vi "Top (FPGA).vi"() -> ()   [LabVIEW 2024, in "PXIe-7903 Aurora Example.lvlib"]
uses:
  PXIe-7903 Aurora Example.lvlib
  <vilib>/Platform/TimedLoop/XDataNode/wakeup.ctl
  <vilib>/Platform/TimedLoop/XDataNode/XDNodeRunTimeDep.lvlib
  <vilib>/Platform/TimedLoop/XDataNode/nitl_modes.ctl
  <vilib>/Platform/TimedLoop/XDataNode/timing_clust.ctl
  <vilib>/Platform/TimedLoop/XDataNode/XDataNode.xnode
  <instrlib>/_niInstr/FIFO Register Bus/v1/FPGA/niInstr FIFO Register Bus v1 FPGA.lvclass
  <instrlib>/_niInstr/Instruction Framework/v1/FPGA/Top Level Bus/Register Configuration/Register Configuration.lvclass
  <instrlib>/_niInstr/Instruction Framework/v1/FPGA/Collection Builder/Collection Builder.lvclass
  <instrlib>/_niInstr/Instruction Framework/v1/FPGA/Collection Builder/Parent Metadata.ctl
  <instrlib>/_niInstr/Instruction Framework/v1/FPGA/Collection Builder/niInstr Address Space Collection Builder v1 FPGA.lvlib
  <vilib>/eio/EIONode/EIONode.xnode
  Utilities/FPGA/Aurora64b66b Utilities FPGA.lvlib
  <instrlib>/_niInstr/Basic Elements/v1/FPGA/niInstr Basic Elements v1 FPGA.lvlib
  <vilib>/rvi/eio/common/nirviEmuTemplateMethod_errors.vi
  <instrlib>/_niInstr/Aurora64b66b/v1/FPGA/Buffered/Aurora64b66b Buffered.lvclass
panel:
  in  "port 11 enable":bool
  in  "port 10 enable":bool
  in  "port 9 enable":bool
  in  "port 8 enable":bool
  in  "port 7 enable":bool
  in  "port 6 enable":bool
  in  "port 5 enable":bool
  in  "port 4 enable":bool
  in  "port 3 enable":bool
  in  "port 2 enable":bool
  in  "port 1 enable":bool
  in  "port 0 enable":bool
  in  "port 11 rx throttle":u16
  out "port 11 mismatch count":u64
  in  "port 10 rx throttle":u16
  out "port 10 mismatch count":u64
  in  "port 9 rx throttle":u16
  out "port 9 mismatch count":u64
  in  "port 8 rx throttle":u16
  out "port 8 mismatch count":u64
  in  "port 7 rx throttle":u16
  out "port 7 mismatch count":u64
  in  "port 6 rx throttle":u16
  out "port 6 mismatch count":u64
  in  "port 5 rx throttle":u16
  out "port 5 mismatch count":u64
  in  "port 4 rx throttle":u16
  out "port 4 mismatch count":u64
  in  "port 3 rx throttle":u16
  out "port 3 mismatch count":u64
  in  "port 2 rx throttle":u16
  out "port 2 mismatch count":u64
  in  "port 1 rx throttle":u16
  out "port 1 mismatch count":u64
  out "port 0 mismatch count":u64
  in  "port 0 rx throttle":u16
  in  "tb reset":bool
  out "flexrio.module.io error 0":i32
  out "flexrio.module.io ready 0":bool
  in  "fifo reg bus ctrl 0":u32
  out "fifo reg bus status 0":u32
  out "fifo reg bus data 0":u64
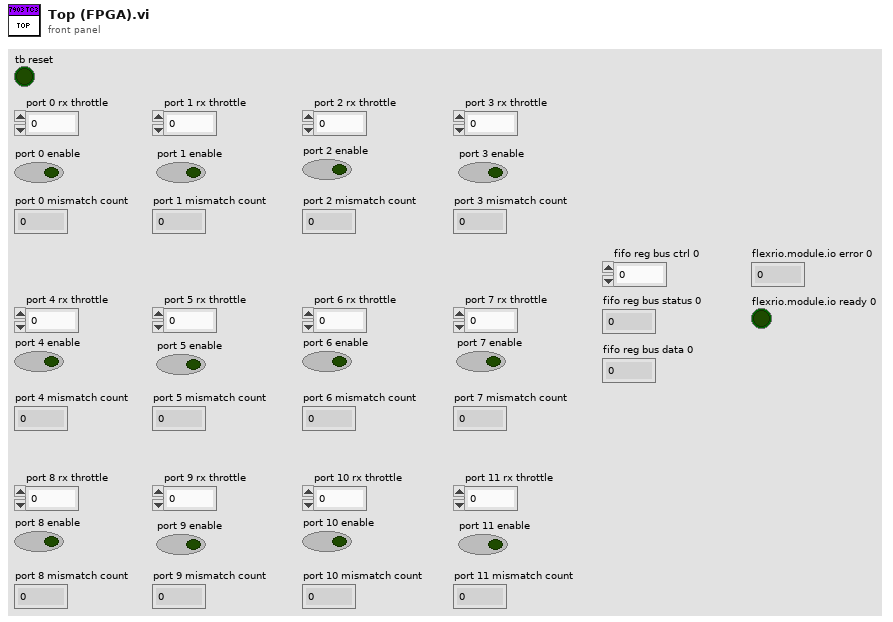
[diagram p1: front panel]
types:
  T1 = typedef "niInstr Address Space Collection Builder v1 FPGA.lvlib/Parent Metadata.ctl" = cluster{"UID":u16, "version":u16, "oldest compatible version":u16}
  T2 = typedef "XDNodeRunTimeDep.lvlib/timing_clust.ctl" = cluster{"Expected End [f-1]":u64, "Actual End [f-1]":u64, "Finished Late? [f-1]":bool, "Expected End [i-1]":u64, "Actual End [i-1]":u64, "Finished Late? [i-1]":bool, "Expected Start [i]":u64, "Actual Start [i]":u64, "Expected Start [f]":u64, "Actual Start [f]":u64, "Source Name":string, "Structure Name":string, "Period":i64, "Deadline":i64, "Offset":i64, "Start":i64, "Priority":i32, "Timeout":i32, "Mode":T3, "Wakeup Reason":T4, "Error":errorcluster, "Source Type":string, "Secondary Source Type":string, "Global End Time":u64, "Global Start Time":u64, "Frame Duration":u64, "Iteration Duration":u64, "Assigned CPU":i32, "I/O Scan Engine Mode":u32}
  T3 = typedef "XDNodeRunTimeDep.lvlib/nitl_modes.ctl" = enum32{"No Change", "Process missed periods, maintain original phase", "Discard missed periods, maintain original phase", "Process missed periods, ignore original phase", "Discard missed periods, ignore original phase"}
  T4 = typedef "XDNodeRunTimeDep.lvlib/wakeup.ctl" = enum32{"Normal", "Aborted", "Asynchronous wakeup", "Timing source error", "Timed loop error", "Timeout"}
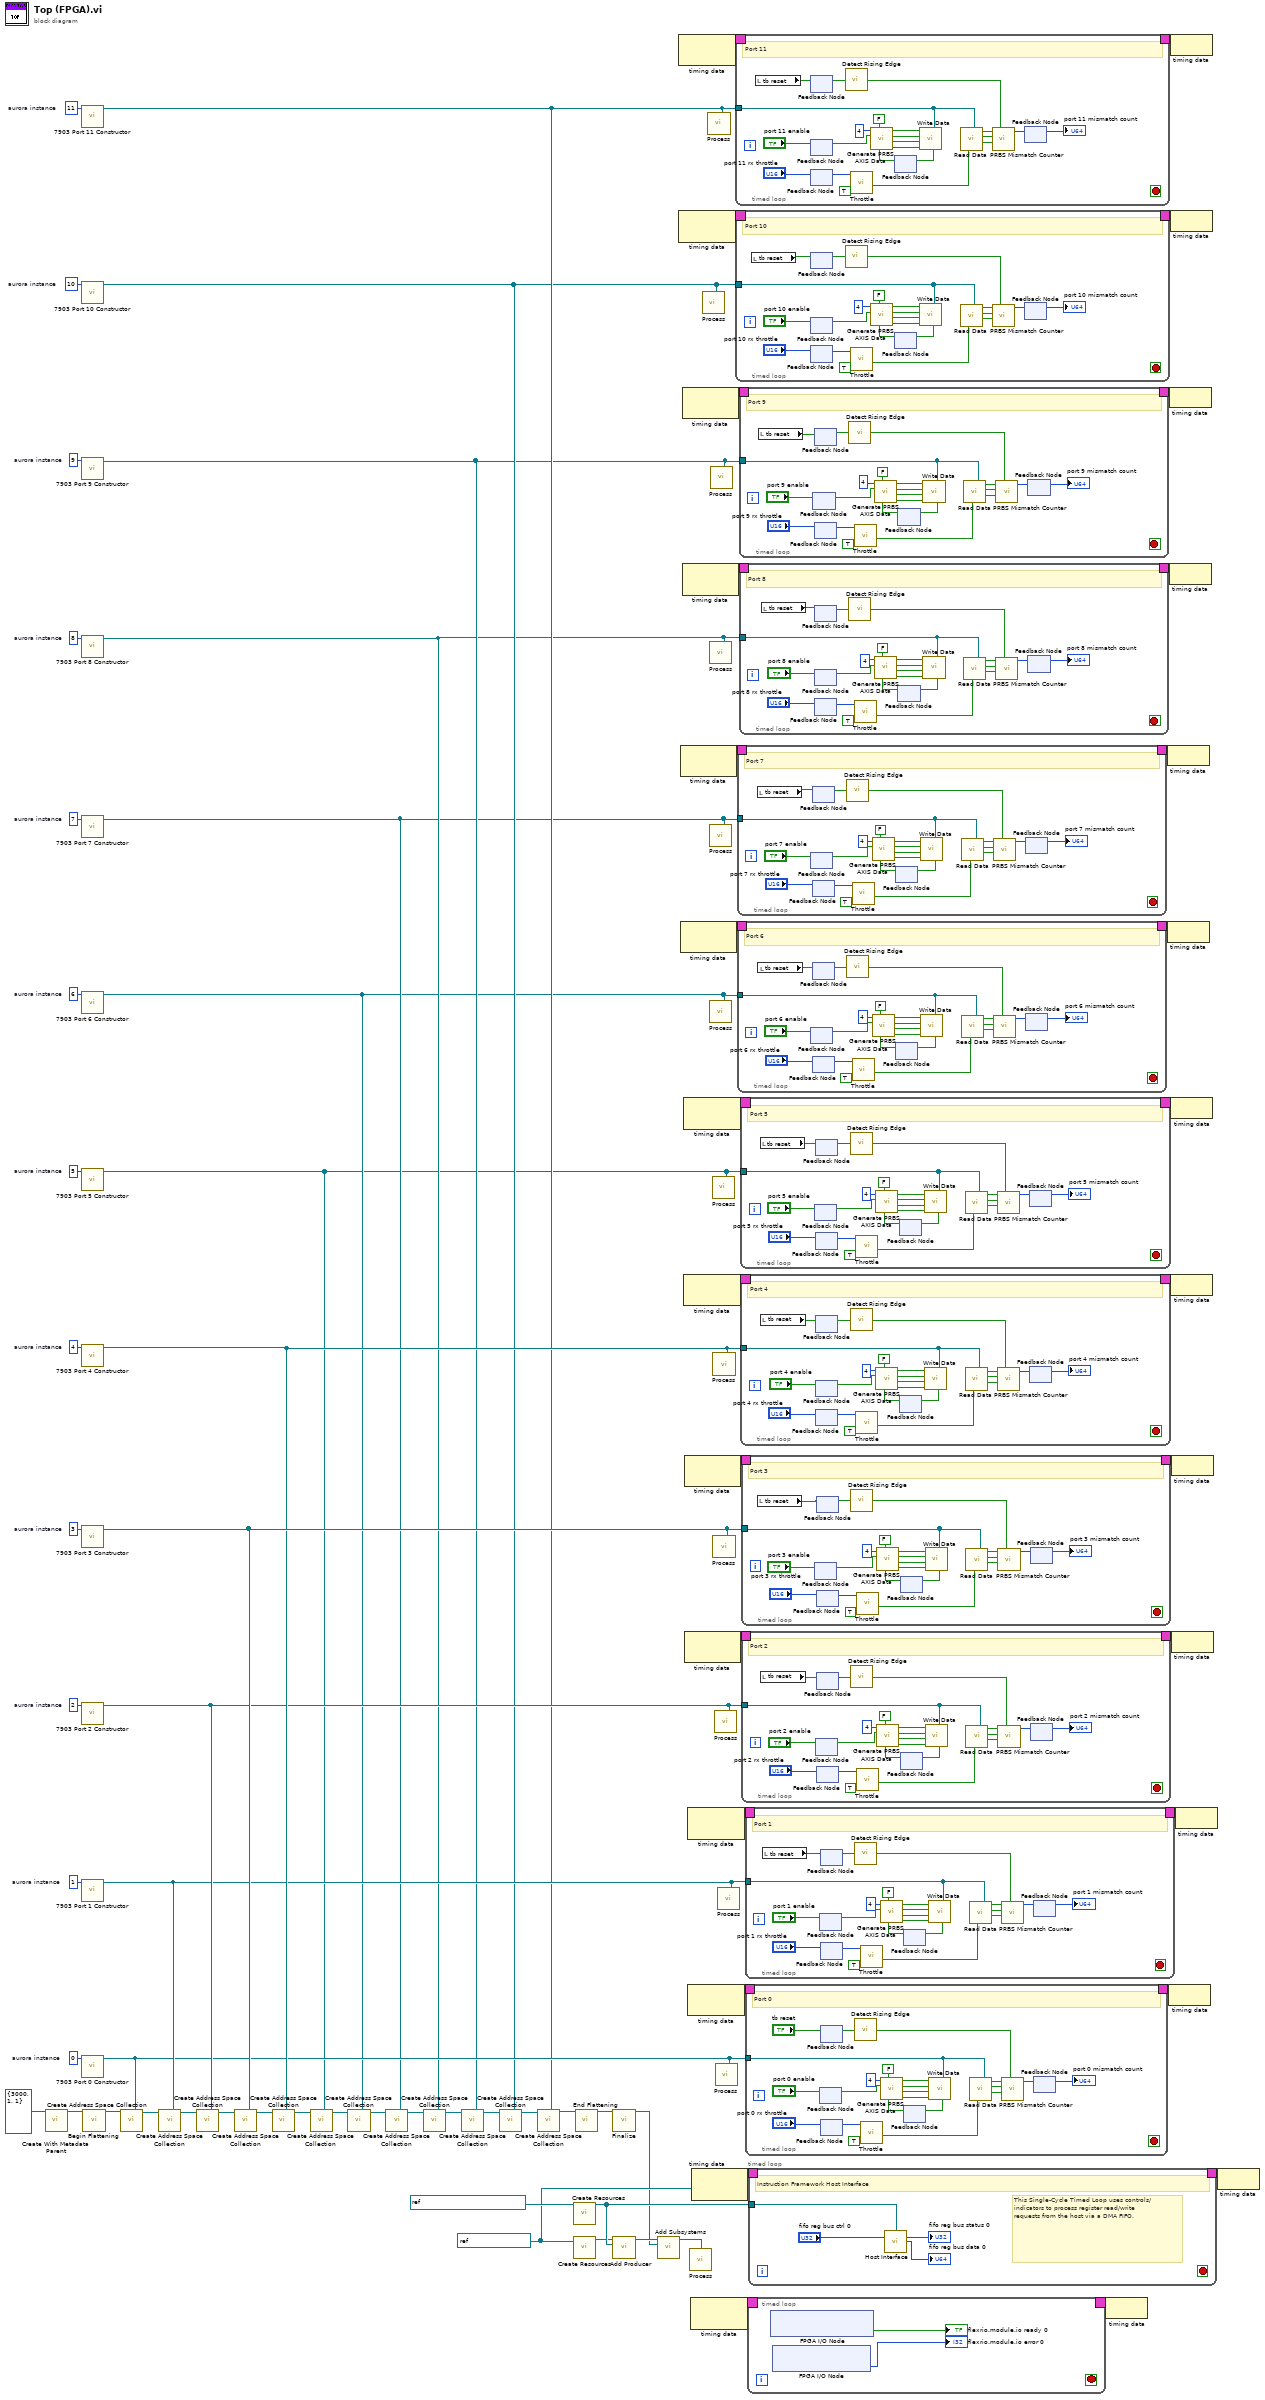
[diagram p0: block diagram]
diagram:
  w1 = u8 11  # aurora instance
  w48 = u8 10  # aurora instance
  w49 = u8 9  # aurora instance
  w50 = u8 8  # aurora instance
  w51 = u8 3  # aurora instance
  w52 = u8 2  # aurora instance
  w53 = u8 1  # aurora instance
  w54 = u8 0  # aurora instance
  w56 = u8 7  # aurora instance
  w57 = u8 6  # aurora instance
  w58 = u8 5  # aurora instance
  w59 = u8 4  # aurora instance
  w70 = refnum<k21> "80 MHz Clock" ("Source Name")
  n1 = call <instrlib>:"Create With Metadata Parent.vi"("parent metadata"=T1 {"UID"=3000, "version"=1, "oldest compatible version"=1}) -> ("collection builder"=w69:refnum<class "Collection Builder.lvclass">)  [unwired: 14 in]
  n2 = call "7903 Port 11 Constructor.vi"("aurora instance (0)"=w1) -> ("aurora64b66b buffered"=w8:refnum<class "Aurora64b66b Buffered.lvclass">)  [unwired: 10 in]
  n3 = call "7903 Port 10 Constructor.vi"("aurora instance (0)"=w48) -> ("aurora64b66b buffered"=w7:refnum<class "Aurora64b66b Buffered.lvclass">)  [unwired: 10 in]
  n4 = call "7903 Port 9 Constructor.vi"("aurora instance (0)"=w49) -> ("aurora64b66b buffered"=w6:refnum<class "Aurora64b66b Buffered.lvclass">)  [unwired: 10 in]
  n5 = call "7903 Port 8 Constructor.vi"("aurora instance (0)"=w50) -> ("aurora64b66b buffered"=w5:refnum<class "Aurora64b66b Buffered.lvclass">)  [unwired: 10 in]
  n6 = call "7903 Port 7 Constructor.vi"("aurora instance (0)"=w56) -> ("aurora64b66b buffered"=w4:refnum<class "Aurora64b66b Buffered.lvclass">)  [unwired: 10 in]
  n7 = call "7903 Port 6 Constructor.vi"("aurora instance (0)"=w57) -> ("aurora64b66b buffered"=w3:refnum<class "Aurora64b66b Buffered.lvclass">)  [unwired: 10 in]
  n8 = call "7903 Port 5 Constructor.vi"("aurora instance (0)"=w58) -> ("aurora64b66b buffered"=w2:refnum<class "Aurora64b66b Buffered.lvclass">)  [unwired: 10 in]
  n9 = call "7903 Port 4 Constructor.vi"("aurora instance (0)"=w59) -> ("aurora64b66b buffered"=w12:refnum<class "Aurora64b66b Buffered.lvclass">)  [unwired: 10 in]
  n10 = call "7903 Port 3 Constructor.vi"("aurora instance (0)"=w51) -> ("aurora64b66b buffered"=w13:refnum<class "Aurora64b66b Buffered.lvclass">)  [unwired: 10 in]
  n11 = call "7903 Port 2 Constructor.vi"("aurora instance (0)"=w52) -> ("aurora64b66b buffered"=w11:refnum<class "Aurora64b66b Buffered.lvclass">)  [unwired: 10 in]
  n12 = call "7903 Port 1 Constructor.vi"("aurora instance (0)"=w53) -> ("aurora64b66b buffered"=w10:refnum<class "Aurora64b66b Buffered.lvclass">)  [unwired: 10 in]
  n13 = call "7903 Port 0 Constructor.vi"("aurora instance (0)"=w54) -> ("aurora64b66b buffered"=w9:refnum<class "Aurora64b66b Buffered.lvclass">)  [unwired: 10 in]
  n14 = call <instrlib>:"Begin Flattening.vi"("collection builder in"=w69) -> ("collection builder out"=w63:refnum<class "Collection Builder.lvclass">)  [unwired: 14 in]
  n15 = call-dynamic "Create Address Space Collection.vi"("aurora64b66b basic"=w9, "collection builder in"=w63) -> ("collection builder out"=w55:refnum<class "Collection Builder.lvclass">)  [unwired: 9 in]
  n16 = call-dynamic "Create Address Space Collection.vi"("aurora64b66b basic"=w10, "collection builder in"=w55) -> ("collection builder out"=w41:refnum<class "Collection Builder.lvclass">)  [unwired: 9 in]
  n17 = call-dynamic "Create Address Space Collection.vi"("aurora64b66b basic"=w11, "collection builder in"=w41) -> ("collection builder out"=w42:refnum<class "Collection Builder.lvclass">)  [unwired: 9 in]
  n18 = call-dynamic "Create Address Space Collection.vi"("aurora64b66b basic"=w13, "collection builder in"=w42) -> ("collection builder out"=w47:refnum<class "Collection Builder.lvclass">)  [unwired: 9 in]
  n19 = call-dynamic "Create Address Space Collection.vi"("aurora64b66b basic"=w12, "collection builder in"=w47) -> ("collection builder out"=w46:refnum<class "Collection Builder.lvclass">)  [unwired: 9 in]
  n20 = call-dynamic "Create Address Space Collection.vi"("aurora64b66b basic"=w2, "collection builder in"=w46) -> ("collection builder out"=w45:refnum<class "Collection Builder.lvclass">)  [unwired: 9 in]
  n21 = call-dynamic "Create Address Space Collection.vi"("aurora64b66b basic"=w3, "collection builder in"=w45) -> ("collection builder out"=w44:refnum<class "Collection Builder.lvclass">)  [unwired: 9 in]
  n22 = call-dynamic "Create Address Space Collection.vi"("aurora64b66b basic"=w4, "collection builder in"=w44) -> ("collection builder out"=w43:refnum<class "Collection Builder.lvclass">)  [unwired: 9 in]
  n23 = call-dynamic "Create Address Space Collection.vi"("aurora64b66b basic"=w5, "collection builder in"=w43) -> ("collection builder out"=w38:refnum<class "Collection Builder.lvclass">)  [unwired: 9 in]
  n24 = call-dynamic "Create Address Space Collection.vi"("aurora64b66b basic"=w6, "collection builder in"=w38) -> ("collection builder out"=w40:refnum<class "Collection Builder.lvclass">)  [unwired: 9 in]
  n25 = call-dynamic "Create Address Space Collection.vi"("aurora64b66b basic"=w7, "collection builder in"=w40) -> ("collection builder out"=w39:refnum<class "Collection Builder.lvclass">)  [unwired: 9 in]
  n26 = call-dynamic "Create Address Space Collection.vi"("aurora64b66b basic"=w8, "collection builder in"=w39) -> ("collection builder out"=w60:refnum<class "Collection Builder.lvclass">)  [unwired: 9 in]
  n27 = call <instrlib>:"Create Resources.vi"("instruction fifo"=refnum<k21> "reg.host instruction fifo 0" ("FIFO")) -> ("fifo register bus"=w72:refnum<class "niInstr FIFO Register Bus v1 FPGA.lvclass">)  [unwired: 14 in]
  n28 = call <instrlib>:"Create Resources.vi"("register clock"=w70) -> ("register configuration"=w71:refnum<class "Register Configuration.lvclass">)  [unwired: 14 in]
  n29 = call <instrlib>:"End Flattening.vi"("collection builder in"=w60) -> ("collection builder out"=w68:refnum<class "Collection Builder.lvclass">)  [unwired: 14 in]
  n30 = call <instrlib>:"Finalize.vi"("collection builder in"=w68) -> ("address space collection"=w64:refnum<class "Address Space Collection.lvclass">)  [unwired: 14 in]
  n31 = call-dynamic "Add Producer.vi"("register configuration in"=w71, "instruction producer"=w72) -> ("register configuration out"=w66:refnum<class "Register Configuration.lvclass">)  [unwired: 13 in]
  n32 = call-dynamic "Add Subsystems.vi"("register configuration in"=w66, "subsystems"=w64) -> ("register configuration out"=w65:refnum<class "Register Configuration.lvclass">)  [unwired: 13 in]
  n33 = node-c288() -> (w15:T2)  [unwired: 1 in]
  n34 = node-c288() -> (w17:T2)  [unwired: 1 in]
  n35 = node-c288() -> (w23:T2)  [unwired: 1 in]
  n36 = node-c288() -> (w25:T2)  [unwired: 1 in]
  n37 = node-c288() -> (w19:T2)  [unwired: 1 in]
  n38 = node-c288() -> (w21:T2)  [unwired: 1 in]
  n39 = node-c288() -> (w27:T2)  [unwired: 1 in]
  n40 = node-c288() -> (w29:T2)  [unwired: 1 in]
  n41 = node-c288() -> (w31:T2)  [unwired: 1 in]
  n42 = node-c288() -> (w33:T2)  [unwired: 1 in]
  n43 = node-c288() -> (w35:T2)  [unwired: 1 in]
  n44 = node-c288() -> (w37:T2)  [unwired: 1 in]
  n45 = call-dynamic "Process.vi"("register configuration"=w65) -> ()  [unwired: 15 in]
  n46 = node-c288() -> (w62:T2)  [unwired: 1 in]
  n47 = node-c288(w70) -> (w75:T2)
  n48 = call-dynamic "Process.vi"("aurora64b66b buffered"=w7) -> ()  [unwired: 11 in]
  n49 = call-dynamic "Process.vi"("aurora64b66b buffered"=w8) -> ()  [unwired: 11 in]
  n50 = call-dynamic "Process.vi"("aurora64b66b buffered"=w5) -> ()  [unwired: 11 in]
  n51 = call-dynamic "Process.vi"("aurora64b66b buffered"=w4) -> ()  [unwired: 11 in]
  n52 = call-dynamic "Process.vi"("aurora64b66b buffered"=w3) -> ()  [unwired: 11 in]
  n53 = call-dynamic "Process.vi"("aurora64b66b buffered"=w6) -> ()  [unwired: 11 in]
  n54 = call-dynamic "Process.vi"("aurora64b66b buffered"=w2) -> ()  [unwired: 11 in]
  n55 = call-dynamic "Process.vi"("aurora64b66b buffered"=w12) -> ()  [unwired: 11 in]
  n56 = call-dynamic "Process.vi"("aurora64b66b buffered"=w13) -> ()  [unwired: 11 in]
  n57 = call-dynamic "Process.vi"("aurora64b66b buffered"=w11) -> ()  [unwired: 11 in]
  n58 = call-dynamic "Process.vi"("aurora64b66b buffered"=w9) -> ()  [unwired: 11 in]
  n59 = call-dynamic "Process.vi"("aurora64b66b buffered"=w10) -> ()  [unwired: 11 in]
  n60 = timed-loop {
    timing: w15 -> [_]
    timing-out: [_] -> w14
    tunnel: w8 -> [w81]
    stop <- _ stop-if-true
    # "Port 11"
    n61 = local read "tb reset"() -> (w79:bool)
    n62 = feedback #1() -> (w76:bool)  [unwired: 1 in]
    n63 = feedback-in #1("port 11 enable") -> ()
    n64 = feedback-in #2(w79) -> ()
    n65 = feedback #2() -> (w82:bool)  [unwired: 1 in]
    n66 = feedback #3() -> (w84:u16)  [unwired: 1 in]
    n67 = feedback-in #3("port 11 rx throttle") -> ()
    n68 = call <instrlib>:"Detect Rising Edge.vi"("signal"=w82) -> ("edge detected"=w96:bool)  [unwired: 14 in]
    n69 = call "Throttle.vi"("request data"=TRUE ("Request Data"), "throttle"=w84) -> ("throttled request"=w89:bool)  [unwired: 9 in]
    n70 = feedback #4() -> (w94:bool)  [unwired: 1 in]
    n71 = call "Generate PRBS AXIS Data.vi"("ready for output"=w94, "reset"=FALSE, "enable"=w76, "number of lanes"=u8 4) -> ("tlast"=w90:bool, "tvalid"=w91:bool, "tkeep"=w92:bool[], "tdata"=w93:bool[])  [unwired: 4 in]
    n72 = call-dynamic "Write Data.vi"("aurora64b66b buffered"=w81, "tlast"=w90, "input valid"=w91, "tkeep"=w92, "tdata"=w93) -> ("ready for input"=w95:bool)  [unwired: 6 in]
    n73 = feedback-in #4(w95) -> ()
    n74 = call-dynamic "Read Data.vi"("aurora64b66b buffered"=w81, "ready for output"=w89) -> ("output valid"=w86:bool, "tkeep"=w87:bool[], "tdata"=w88:bool[])  [unwired: 6 in, 1 out]
    n75 = call "PRBS Mismatch Counter.vi"("reset mismatch count"=w96, "input valid"=w86, "tkeep"=w87, "data in"=w88) -> ("mismatch count"=w97:u64)  [unwired: 7 in]
    n76 = feedback-in #5(w97) -> ()
    n77 = feedback #5() -> (→"port 11 mismatch count":u64)  [unwired: 1 in]
  }
  n78 = timed-loop {
    timing: w17 -> [_]
    timing-out: [_] -> w16
    tunnel: w7 -> [w106]
    stop <- _ stop-if-true
    # "Port 10"
    n79 = local read "tb reset"() -> (w104:bool)
    n80 = feedback #6() -> (w101:bool)  [unwired: 1 in]
    n81 = feedback-in #6("port 10 enable") -> ()
    n82 = feedback-in #7(w104) -> ()
    n83 = feedback #7() -> (w107:bool)  [unwired: 1 in]
    n84 = feedback #8() -> (w109:u16)  [unwired: 1 in]
    n85 = feedback-in #8("port 10 rx throttle") -> ()
    n86 = call <instrlib>:"Detect Rising Edge.vi"("signal"=w107) -> ("edge detected"=w121:bool)  [unwired: 14 in]
    n87 = call "Throttle.vi"("request data"=TRUE ("Request Data"), "throttle"=w109) -> ("throttled request"=w114:bool)  [unwired: 9 in]
    n88 = feedback #9() -> (w119:bool)  [unwired: 1 in]
    n89 = call "Generate PRBS AXIS Data.vi"("ready for output"=w119, "reset"=FALSE, "enable"=w101, "number of lanes"=u8 4) -> ("tlast"=w115:bool, "tvalid"=w116:bool, "tkeep"=w117:bool[], "tdata"=w118:bool[])  [unwired: 4 in]
    n90 = call-dynamic "Write Data.vi"("aurora64b66b buffered"=w106, "tlast"=w115, "input valid"=w116, "tkeep"=w117, "tdata"=w118) -> ("ready for input"=w120:bool)  [unwired: 6 in]
    n91 = feedback-in #9(w120) -> ()
    n92 = call-dynamic "Read Data.vi"("aurora64b66b buffered"=w106, "ready for output"=w114) -> ("output valid"=w111:bool, "tkeep"=w112:bool[], "tdata"=w113:bool[])  [unwired: 6 in, 1 out]
    n93 = call "PRBS Mismatch Counter.vi"("reset mismatch count"=w121, "input valid"=w111, "tkeep"=w112, "data in"=w113) -> ("mismatch count"=w122:u64)  [unwired: 7 in]
    n94 = feedback-in #10(w122) -> ()
    n95 = feedback #10() -> (→"port 10 mismatch count":u64)  [unwired: 1 in]
  }
  n96 = timed-loop {
    timing: w23 -> [_]
    timing-out: [_] -> w22
    tunnel: w4 -> [w131]
    stop <- _ stop-if-true
    # "Port 7"
    n97 = local read "tb reset"() -> (w129:bool)
    n98 = feedback #11() -> (w126:bool)  [unwired: 1 in]
    n99 = feedback-in #11("port 7 enable") -> ()
    n100 = feedback-in #12(w129) -> ()
    n101 = feedback #12() -> (w132:bool)  [unwired: 1 in]
    n102 = feedback #13() -> (w134:u16)  [unwired: 1 in]
    n103 = feedback-in #13("port 7 rx throttle") -> ()
    n104 = call <instrlib>:"Detect Rising Edge.vi"("signal"=w132) -> ("edge detected"=w146:bool)  [unwired: 14 in]
    n105 = call "Throttle.vi"("request data"=TRUE ("Request Data"), "throttle"=w134) -> ("throttled request"=w139:bool)  [unwired: 9 in]
    n106 = feedback #14() -> (w144:bool)  [unwired: 1 in]
    n107 = call "Generate PRBS AXIS Data.vi"("ready for output"=w144, "reset"=FALSE, "enable"=w126, "number of lanes"=u8 4) -> ("tlast"=w140:bool, "tvalid"=w141:bool, "tkeep"=w142:bool[], "tdata"=w143:bool[])  [unwired: 4 in]
    n108 = call-dynamic "Write Data.vi"("aurora64b66b buffered"=w131, "tlast"=w140, "input valid"=w141, "tkeep"=w142, "tdata"=w143) -> ("ready for input"=w145:bool)  [unwired: 6 in]
    n109 = feedback-in #14(w145) -> ()
    n110 = call-dynamic "Read Data.vi"("aurora64b66b buffered"=w131, "ready for output"=w139) -> ("output valid"=w136:bool, "tkeep"=w137:bool[], "tdata"=w138:bool[])  [unwired: 6 in, 1 out]
    n111 = call "PRBS Mismatch Counter.vi"("reset mismatch count"=w146, "input valid"=w136, "tkeep"=w137, "data in"=w138) -> ("mismatch count"=w147:u64)  [unwired: 7 in]
    n112 = feedback-in #15(w147) -> ()
    n113 = feedback #15() -> (→"port 7 mismatch count":u64)  [unwired: 1 in]
  }
  n114 = timed-loop {
    timing: w25 -> [_]
    timing-out: [_] -> w24
    tunnel: w3 -> [w156]
    stop <- _ stop-if-true
    # "Port 6"
    n115 = local read "tb reset"() -> (w154:bool)
    n116 = feedback #16() -> (w151:bool)  [unwired: 1 in]
    n117 = feedback-in #16("port 6 enable") -> ()
    n118 = feedback-in #17(w154) -> ()
    n119 = feedback #17() -> (w157:bool)  [unwired: 1 in]
    n120 = feedback #18() -> (w159:u16)  [unwired: 1 in]
    n121 = feedback-in #18("port 6 rx throttle") -> ()
    n122 = call <instrlib>:"Detect Rising Edge.vi"("signal"=w157) -> ("edge detected"=w171:bool)  [unwired: 14 in]
    n123 = call "Throttle.vi"("request data"=TRUE ("Request Data"), "throttle"=w159) -> ("throttled request"=w164:bool)  [unwired: 9 in]
    n124 = feedback #19() -> (w169:bool)  [unwired: 1 in]
    n125 = call "Generate PRBS AXIS Data.vi"("ready for output"=w169, "reset"=FALSE, "enable"=w151, "number of lanes"=u8 4) -> ("tlast"=w165:bool, "tvalid"=w166:bool, "tkeep"=w167:bool[], "tdata"=w168:bool[])  [unwired: 4 in]
    n126 = call-dynamic "Write Data.vi"("aurora64b66b buffered"=w156, "tlast"=w165, "input valid"=w166, "tkeep"=w167, "tdata"=w168) -> ("ready for input"=w170:bool)  [unwired: 6 in]
    n127 = feedback-in #19(w170) -> ()
    n128 = call-dynamic "Read Data.vi"("aurora64b66b buffered"=w156, "ready for output"=w164) -> ("output valid"=w161:bool, "tkeep"=w162:bool[], "tdata"=w163:bool[])  [unwired: 6 in, 1 out]
    n129 = call "PRBS Mismatch Counter.vi"("reset mismatch count"=w171, "input valid"=w161, "tkeep"=w162, "data in"=w163) -> ("mismatch count"=w172:u64)  [unwired: 7 in]
    n130 = feedback-in #20(w172) -> ()
    n131 = feedback #20() -> (→"port 6 mismatch count":u64)  [unwired: 1 in]
  }
  n132 = timed-loop {
    timing: w19 -> [_]
    timing-out: [_] -> w18
    tunnel: w6 -> [w181]
    stop <- _ stop-if-true
    # "Port 9"
    n133 = local read "tb reset"() -> (w179:bool)
    n134 = feedback #21() -> (w176:bool)  [unwired: 1 in]
    n135 = feedback-in #21("port 9 enable") -> ()
    n136 = feedback-in #22(w179) -> ()
    n137 = feedback #22() -> (w182:bool)  [unwired: 1 in]
    n138 = feedback #23() -> (w184:u16)  [unwired: 1 in]
    n139 = feedback-in #23("port 9 rx throttle") -> ()
    n140 = call <instrlib>:"Detect Rising Edge.vi"("signal"=w182) -> ("edge detected"=w196:bool)  [unwired: 14 in]
    n141 = call "Throttle.vi"("request data"=TRUE ("Request Data"), "throttle"=w184) -> ("throttled request"=w189:bool)  [unwired: 9 in]
    n142 = feedback #24() -> (w194:bool)  [unwired: 1 in]
    n143 = call "Generate PRBS AXIS Data.vi"("ready for output"=w194, "reset"=FALSE, "enable"=w176, "number of lanes"=u8 4) -> ("tlast"=w190:bool, "tvalid"=w191:bool, "tkeep"=w192:bool[], "tdata"=w193:bool[])  [unwired: 4 in]
    n144 = call-dynamic "Write Data.vi"("aurora64b66b buffered"=w181, "tlast"=w190, "input valid"=w191, "tkeep"=w192, "tdata"=w193) -> ("ready for input"=w195:bool)  [unwired: 6 in]
    n145 = feedback-in #24(w195) -> ()
    n146 = call-dynamic "Read Data.vi"("aurora64b66b buffered"=w181, "ready for output"=w189) -> ("output valid"=w186:bool, "tkeep"=w187:bool[], "tdata"=w188:bool[])  [unwired: 6 in, 1 out]
    n147 = call "PRBS Mismatch Counter.vi"("reset mismatch count"=w196, "input valid"=w186, "tkeep"=w187, "data in"=w188) -> ("mismatch count"=w197:u64)  [unwired: 7 in]
    n148 = feedback-in #25(w197) -> ()
    n149 = feedback #25() -> (→"port 9 mismatch count":u64)  [unwired: 1 in]
  }
  n150 = timed-loop {
    timing: w21 -> [_]
    timing-out: [_] -> w20
    tunnel: w5 -> [w206]
    stop <- _ stop-if-true
    # "Port 8"
    n151 = local read "tb reset"() -> (w204:bool)
    n152 = feedback-in #26(w204) -> ()
    n153 = feedback #26() -> (w207:bool)  [unwired: 1 in]
    n154 = feedback #27() -> (w201:bool)  [unwired: 1 in]
    n155 = feedback-in #27("port 8 enable") -> ()
    n156 = feedback #28() -> (w209:u16)  [unwired: 1 in]
    n157 = feedback-in #28("port 8 rx throttle") -> ()
    n158 = call <instrlib>:"Detect Rising Edge.vi"("signal"=w207) -> ("edge detected"=w221:bool)  [unwired: 14 in]
    n159 = call "Throttle.vi"("request data"=TRUE ("Request Data"), "throttle"=w209) -> ("throttled request"=w214:bool)  [unwired: 9 in]
    n160 = feedback #29() -> (w219:bool)  [unwired: 1 in]
    n161 = call "Generate PRBS AXIS Data.vi"("ready for output"=w219, "reset"=FALSE, "enable"=w201, "number of lanes"=u8 4) -> ("tlast"=w215:bool, "tvalid"=w216:bool, "tkeep"=w217:bool[], "tdata"=w218:bool[])  [unwired: 4 in]
    n162 = call-dynamic "Write Data.vi"("aurora64b66b buffered"=w206, "tlast"=w215, "input valid"=w216, "tkeep"=w217, "tdata"=w218) -> ("ready for input"=w220:bool)  [unwired: 6 in]
    n163 = feedback-in #29(w220) -> ()
    n164 = call-dynamic "Read Data.vi"("aurora64b66b buffered"=w206, "ready for output"=w214) -> ("output valid"=w211:bool, "tkeep"=w212:bool[], "tdata"=w213:bool[])  [unwired: 6 in, 1 out]
    n165 = call "PRBS Mismatch Counter.vi"("reset mismatch count"=w221, "input valid"=w211, "tkeep"=w212, "data in"=w213) -> ("mismatch count"=w222:u64)  [unwired: 7 in]
    n166 = feedback-in #30(w222) -> ()
    n167 = feedback #30() -> (→"port 8 mismatch count":u64)  [unwired: 1 in]
  }
  n168 = timed-loop {
    timing: w27 -> [_]
    timing-out: [_] -> w26
    tunnel: w2 -> [w231]
    stop <- _ stop-if-true
    # "Port 5"
    n169 = local read "tb reset"() -> (w229:bool)
    n170 = feedback #31() -> (w226:bool)  [unwired: 1 in]
    n171 = feedback-in #31("port 5 enable") -> ()
    n172 = feedback-in #32(w229) -> ()
    n173 = feedback #32() -> (w232:bool)  [unwired: 1 in]
    n174 = feedback #33() -> (w234:u16)  [unwired: 1 in]
    n175 = feedback-in #33("port 5 rx throttle") -> ()
    n176 = call <instrlib>:"Detect Rising Edge.vi"("signal"=w232) -> ("edge detected"=w246:bool)  [unwired: 14 in]
    n177 = call "Throttle.vi"("request data"=TRUE ("Request Data"), "throttle"=w234) -> ("throttled request"=w239:bool)  [unwired: 9 in]
    n178 = feedback #34() -> (w244:bool)  [unwired: 1 in]
    n179 = call "Generate PRBS AXIS Data.vi"("ready for output"=w244, "reset"=FALSE, "enable"=w226, "number of lanes"=u8 4) -> ("tlast"=w240:bool, "tvalid"=w241:bool, "tkeep"=w242:bool[], "tdata"=w243:bool[])  [unwired: 4 in]
    n180 = call-dynamic "Write Data.vi"("aurora64b66b buffered"=w231, "tlast"=w240, "input valid"=w241, "tkeep"=w242, "tdata"=w243) -> ("ready for input"=w245:bool)  [unwired: 6 in]
    n181 = feedback-in #34(w245) -> ()
    n182 = call-dynamic "Read Data.vi"("aurora64b66b buffered"=w231, "ready for output"=w239) -> ("output valid"=w236:bool, "tkeep"=w237:bool[], "tdata"=w238:bool[])  [unwired: 6 in, 1 out]
    n183 = call "PRBS Mismatch Counter.vi"("reset mismatch count"=w246, "input valid"=w236, "tkeep"=w237, "data in"=w238) -> ("mismatch count"=w247:u64)  [unwired: 7 in]
    n184 = feedback-in #35(w247) -> ()
    n185 = feedback #35() -> (→"port 5 mismatch count":u64)  [unwired: 1 in]
  }
  n186 = timed-loop {
    timing: w29 -> [_]
    timing-out: [_] -> w28
    tunnel: w12 -> [w256]
    stop <- _ stop-if-true
    # "Port 4"
    n187 = local read "tb reset"() -> (w254:bool)
    n188 = feedback-in #36(w254) -> ()
    n189 = feedback #36() -> (w257:bool)  [unwired: 1 in]
    n190 = feedback #37() -> (w251:bool)  [unwired: 1 in]
    n191 = feedback-in #37("port 4 enable") -> ()
    n192 = feedback #38() -> (w259:u16)  [unwired: 1 in]
    n193 = feedback-in #38("port 4 rx throttle") -> ()
    n194 = call <instrlib>:"Detect Rising Edge.vi"("signal"=w257) -> ("edge detected"=w271:bool)  [unwired: 14 in]
    n195 = call "Throttle.vi"("request data"=TRUE ("Request Data"), "throttle"=w259) -> ("throttled request"=w264:bool)  [unwired: 9 in]
    n196 = feedback #39() -> (w269:bool)  [unwired: 1 in]
    n197 = call "Generate PRBS AXIS Data.vi"("ready for output"=w269, "reset"=FALSE, "enable"=w251, "number of lanes"=u8 4) -> ("tlast"=w265:bool, "tvalid"=w266:bool, "tkeep"=w267:bool[], "tdata"=w268:bool[])  [unwired: 4 in]
    n198 = call-dynamic "Write Data.vi"("aurora64b66b buffered"=w256, "tlast"=w265, "input valid"=w266, "tkeep"=w267, "tdata"=w268) -> ("ready for input"=w270:bool)  [unwired: 6 in]
    n199 = feedback-in #39(w270) -> ()
    n200 = call-dynamic "Read Data.vi"("aurora64b66b buffered"=w256, "ready for output"=w264) -> ("output valid"=w261:bool, "tkeep"=w262:bool[], "tdata"=w263:bool[])  [unwired: 6 in, 1 out]
    n201 = call "PRBS Mismatch Counter.vi"("reset mismatch count"=w271, "input valid"=w261, "tkeep"=w262, "data in"=w263) -> ("mismatch count"=w272:u64)  [unwired: 7 in]
    n202 = feedback-in #40(w272) -> ()
    n203 = feedback #40() -> (→"port 4 mismatch count":u64)  [unwired: 1 in]
  }
  n204 = timed-loop {
    timing: w31 -> [_]
    timing-out: [_] -> w30
    tunnel: w13 -> [w281]
    stop <- _ stop-if-true
    # "Port 3"
    n205 = local read "tb reset"() -> (w279:bool)
    n206 = feedback #41() -> (w276:bool)  [unwired: 1 in]
    n207 = feedback-in #41("port 3 enable") -> ()
    n208 = feedback-in #42(w279) -> ()
    n209 = feedback #42() -> (w282:bool)  [unwired: 1 in]
    n210 = feedback #43() -> (w284:u16)  [unwired: 1 in]
    n211 = feedback-in #43("port 3 rx throttle") -> ()
    n212 = call <instrlib>:"Detect Rising Edge.vi"("signal"=w282) -> ("edge detected"=w296:bool)  [unwired: 14 in]
    n213 = call "Throttle.vi"("request data"=TRUE ("Request Data"), "throttle"=w284) -> ("throttled request"=w289:bool)  [unwired: 9 in]
    n214 = feedback #44() -> (w294:bool)  [unwired: 1 in]
    n215 = call "Generate PRBS AXIS Data.vi"("ready for output"=w294, "reset"=FALSE, "enable"=w276, "number of lanes"=u8 4) -> ("tlast"=w290:bool, "tvalid"=w291:bool, "tkeep"=w292:bool[], "tdata"=w293:bool[])  [unwired: 4 in]
    n216 = call-dynamic "Write Data.vi"("aurora64b66b buffered"=w281, "tlast"=w290, "input valid"=w291, "tkeep"=w292, "tdata"=w293) -> ("ready for input"=w295:bool)  [unwired: 6 in]
    n217 = feedback-in #44(w295) -> ()
    n218 = call-dynamic "Read Data.vi"("aurora64b66b buffered"=w281, "ready for output"=w289) -> ("output valid"=w286:bool, "tkeep"=w287:bool[], "tdata"=w288:bool[])  [unwired: 6 in, 1 out]
    n219 = call "PRBS Mismatch Counter.vi"("reset mismatch count"=w296, "input valid"=w286, "tkeep"=w287, "data in"=w288) -> ("mismatch count"=w297:u64)  [unwired: 7 in]
    n220 = feedback-in #45(w297) -> ()
    n221 = feedback #45() -> (→"port 3 mismatch count":u64)  [unwired: 1 in]
  }
  n222 = timed-loop {
    timing: w33 -> [_]
    timing-out: [_] -> w32
    tunnel: w11 -> [w306]
    stop <- _ stop-if-true
    # "Port 2"
    n223 = local read "tb reset"() -> (w304:bool)
    n224 = feedback #46() -> (w301:bool)  [unwired: 1 in]
    n225 = feedback-in #46("port 2 enable") -> ()
    n226 = feedback-in #47(w304) -> ()
    n227 = feedback #47() -> (w307:bool)  [unwired: 1 in]
    n228 = feedback #48() -> (w309:u16)  [unwired: 1 in]
    n229 = feedback-in #48("port 2 rx throttle") -> ()
    n230 = call <instrlib>:"Detect Rising Edge.vi"("signal"=w307) -> ("edge detected"=w321:bool)  [unwired: 14 in]
    n231 = call "Throttle.vi"("request data"=TRUE ("Request Data"), "throttle"=w309) -> ("throttled request"=w314:bool)  [unwired: 9 in]
    n232 = feedback #49() -> (w319:bool)  [unwired: 1 in]
    n233 = call "Generate PRBS AXIS Data.vi"("ready for output"=w319, "reset"=FALSE, "enable"=w301, "number of lanes"=u8 4) -> ("tlast"=w315:bool, "tvalid"=w316:bool, "tkeep"=w317:bool[], "tdata"=w318:bool[])  [unwired: 4 in]
    n234 = call-dynamic "Write Data.vi"("aurora64b66b buffered"=w306, "tlast"=w315, "input valid"=w316, "tkeep"=w317, "tdata"=w318) -> ("ready for input"=w320:bool)  [unwired: 6 in]
    n235 = feedback-in #49(w320) -> ()
    n236 = call-dynamic "Read Data.vi"("aurora64b66b buffered"=w306, "ready for output"=w314) -> ("output valid"=w311:bool, "tkeep"=w312:bool[], "tdata"=w313:bool[])  [unwired: 6 in, 1 out]
    n237 = call "PRBS Mismatch Counter.vi"("reset mismatch count"=w321, "input valid"=w311, "tkeep"=w312, "data in"=w313) -> ("mismatch count"=w322:u64)  [unwired: 7 in]
    n238 = feedback-in #50(w322) -> ()
    n239 = feedback #50() -> (→"port 2 mismatch count":u64)  [unwired: 1 in]
  }
  n240 = timed-loop {
    timing: w35 -> [_]
    timing-out: [_] -> w34
    tunnel: w10 -> [w331]
    stop <- _ stop-if-true
    # "Port 1"
    n241 = local read "tb reset"() -> (w329:bool)
    n242 = feedback #51() -> (w326:bool)  [unwired: 1 in]
    n243 = feedback-in #51("port 1 enable") -> ()
    n244 = feedback-in #52(w329) -> ()
    n245 = feedback #52() -> (w332:bool)  [unwired: 1 in]
    n246 = feedback #53() -> (w334:u16)  [unwired: 1 in]
    n247 = feedback-in #53("port 1 rx throttle") -> ()
    n248 = call <instrlib>:"Detect Rising Edge.vi"("signal"=w332) -> ("edge detected"=w346:bool)  [unwired: 14 in]
    n249 = call "Throttle.vi"("request data"=TRUE ("Request Data"), "throttle"=w334) -> ("throttled request"=w339:bool)  [unwired: 9 in]
    n250 = feedback #54() -> (w344:bool)  [unwired: 1 in]
    n251 = call "Generate PRBS AXIS Data.vi"("ready for output"=w344, "reset"=FALSE, "enable"=w326, "number of lanes"=u8 4) -> ("tlast"=w340:bool, "tvalid"=w341:bool, "tkeep"=w342:bool[], "tdata"=w343:bool[])  [unwired: 4 in]
    n252 = call-dynamic "Write Data.vi"("aurora64b66b buffered"=w331, "tlast"=w340, "input valid"=w341, "tkeep"=w342, "tdata"=w343) -> ("ready for input"=w345:bool)  [unwired: 6 in]
    n253 = feedback-in #54(w345) -> ()
    n254 = call-dynamic "Read Data.vi"("aurora64b66b buffered"=w331, "ready for output"=w339) -> ("output valid"=w336:bool, "tkeep"=w337:bool[], "tdata"=w338:bool[])  [unwired: 6 in, 1 out]
    n255 = call "PRBS Mismatch Counter.vi"("reset mismatch count"=w346, "input valid"=w336, "tkeep"=w337, "data in"=w338) -> ("mismatch count"=w347:u64)  [unwired: 7 in]
    n256 = feedback-in #55(w347) -> ()
    n257 = feedback #55() -> (→"port 1 mismatch count":u64)  [unwired: 1 in]
  }
  n258 = timed-loop {
    timing: w37 -> [_]
    timing-out: [_] -> w36
    tunnel: w9 -> [w355]
    stop <- _ stop-if-true
    # "Port 0"
    n259 = feedback #56() -> (w351:bool)  [unwired: 1 in]
    n260 = feedback-in #56("port 0 enable") -> ()
    n261 = feedback-in #57("tb reset") -> ()
    n262 = feedback #57() -> (w356:bool)  [unwired: 1 in]
    n263 = feedback #58() -> (w359:u16)  [unwired: 1 in]
    n264 = feedback-in #58("port 0 rx throttle") -> ()
    n265 = call <instrlib>:"Detect Rising Edge.vi"("signal"=w356) -> ("edge detected"=w371:bool)  [unwired: 14 in]
    n266 = call "Throttle.vi"("request data"=TRUE ("Request Data"), "throttle"=w359) -> ("throttled request"=w364:bool)  [unwired: 9 in]
    n267 = feedback #59() -> (w369:bool)  [unwired: 1 in]
    n268 = call "Generate PRBS AXIS Data.vi"("ready for output"=w369, "reset"=FALSE, "enable"=w351, "number of lanes"=u8 4) -> ("tlast"=w365:bool, "tvalid"=w366:bool, "tkeep"=w367:bool[], "tdata"=w368:bool[])  [unwired: 4 in]
    n269 = call-dynamic "Write Data.vi"("aurora64b66b buffered"=w355, "tlast"=w365, "input valid"=w366, "tkeep"=w367, "tdata"=w368) -> ("ready for input"=w370:bool)  [unwired: 6 in]
    n270 = feedback-in #59(w370) -> ()
    n271 = call-dynamic "Read Data.vi"("aurora64b66b buffered"=w355, "ready for output"=w364) -> ("output valid"=w361:bool, "tkeep"=w362:bool[], "tdata"=w363:bool[])  [unwired: 6 in, 1 out]
    n272 = call "PRBS Mismatch Counter.vi"("reset mismatch count"=w371, "input valid"=w361, "tkeep"=w362, "data in"=w363) -> ("mismatch count"=w372:u64)  [unwired: 7 in]
    n273 = feedback-in #60(w372) -> ()
    n274 = feedback #60() -> (→"port 0 mismatch count":u64)  [unwired: 1 in]
  }
  n275 = timed-loop {
    timing: w62 -> [_]
    timing-out: [_] -> w61
    stop <- _ stop-if-true
    n276 = xnode "FPGA I/O Node"() -> ("IO Socket.IO Ready"=→"flexrio.module.io ready 0":bool)  [unwired: 1 in, 1 out]
    n277 = xnode "FPGA I/O Node"() -> ("IO Socket.IO Error"=→"flexrio.module.io error 0":i32)  [unwired: 1 in, 1 out]
  }
  n278 = timed-loop {
    timing: w75 -> [_]
    timing-out: [_] -> w74
    tunnel: w72 -> [w380]
    stop <- _ stop-if-true
    # "This Single-Cycle Timed Loop uses controls/indicators to process register read/write requests from the host via a DMA FIFO."
    # "Instruction Framework Host Interface"
    n279 = call <instrlib>:"Host Interface.vi"("fifo register bus"=w380, "fifo reg bus ctrl 0"="fifo reg bus ctrl 0") -> ("fifo reg bus status 0"=→"fifo reg bus status 0":u32, "fifo reg bus data 0"=→"fifo reg bus data 0":u64)  [unwired: 12 in]
  }
  n280 = node-c288(w61) -> ()
  n281 = node-c288(w22) -> ()
  n282 = node-c288(w24) -> ()
  n283 = node-c288(w36) -> ()
  n284 = node-c288(w18) -> ()
  n285 = node-c288(w20) -> ()
  n286 = node-c288(w14) -> ()
  n287 = node-c288(w16) -> ()
  n288 = node-c288(w26) -> ()
  n289 = node-c288(w28) -> ()
  n290 = node-c288(w30) -> ()
  n291 = node-c288(w32) -> ()
  n292 = node-c288(w34) -> ()
  n293 = node-c288(w74) -> ()
